vi "Test arcsus comm.vi"() -> ()   [LabVIEW 2012]
uses:
  PerformaxLV_v102.llb/commands.ctl
panel:
  out "Microstep":string
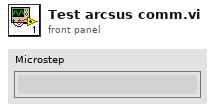
[diagram p1: front panel]
types:
  T1 = typedef "commands.ctl" = enum16{"clearErr", "constJogNeg", "constJogPos", "getAccel", "getDeviceId", "getFirmwareVer", "getHighSpeed", "getIdleAmp", "getLowSpeed", "getMicroStep", "getMotorStatus", "getPolarity", "getPosition", "getProdId", "getPwrStatus", "getRunAmp", "getStatus", "getTemp", "homeNeg", "homePos", "moveToPosition", "powerDown", "powerUp", "setAccel", "setDeviceId", "setHighSpeed", "setIdleAmp", "setLowSpeed", "setMicroStep", "setPolarityLow", "setPolarityHigh", "setPosition", "setRunAmp", "stopFast", "stopSlow"}
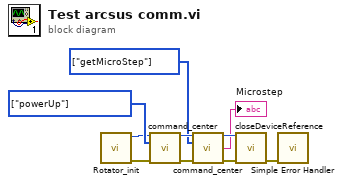
[diagram p0: block diagram]
diagram:
  w5 = T1[] [enum."getMicroStep"] items=["clearErr", "constJogNeg", "constJogPos", "getAccel", "getDeviceId", "getFirmwareVer", "getHighSpeed", "getIdleAmp", "getLowSpeed", "getMicroStep", "getMotorStatus", "getPolarity", "getPosition", "getProdId", "getPwrStatus", "getRunAmp", "getStatus", "getTemp", "homeNeg", "homePos", "moveToPosition", "powerDown", "powerUp", "setAccel", "setDeviceId", "setHighSpeed", "setIdleAmp", "setLowSpeed", "setMicroStep", "setPolarityLow", "setPolarityHigh", "setPosition", "setRunAmp", "stopFast", "stopSlow"] ("commands")
  w9 = T1[] [enum."powerUp"] items=["clearErr", "constJogNeg", "constJogPos", "getAccel", "getDeviceId", "getFirmwareVer", "getHighSpeed", "getIdleAmp", "getLowSpeed", "getMicroStep", "getMotorStatus", "getPolarity", "getPosition", "getProdId", "getPwrStatus", "getRunAmp", "getStatus", "getTemp", "homeNeg", "homePos", "moveToPosition", "powerDown", "powerUp", "setAccel", "setDeviceId", "setHighSpeed", "setIdleAmp", "setLowSpeed", "setMicroStep", "setPolarityLow", "setPolarityHigh", "setPosition", "setRunAmp", "stopFast", "stopSlow"] ("commands")
  n1 = call "Rotator_init.vi"() -> ("error out"=w10:errorcluster, "reference"=w8:i32)  [unwired: 2 in, 8 out]
  n2 = call "command_center.vi"("reference (in)"=w8, "commands"=w9, "error in (no error)"=w10) -> ("reference (out)"=w6:i32, "error out"=w7:errorcluster)  [unwired: 1 in, 10 out]
  n3 = call "command_center.vi"("reference (in)"=w6, "commands"=w5, "error in (no error)"=w7) -> ("reference (out)"=w3:i32, "data (out)"=→"Microstep":string, "error out"=w4:errorcluster)  [unwired: 1 in, 9 out]
  n4 = call "closeDeviceReference.vi"("reference"=w3, "error in (no error)"=w4) -> ("error out"=w1:errorcluster)  [unwired: 1 in, 12 out]
  n5 = call <vilib>:"Simple Error Handler.vi"("error in (no error)"=w1) -> ()  [unwired: 4 in, 5 out]
